vi "Helper Methods Launcher.vi"() -> ()   [LabVIEW 2020, in "2. Basic Panel Actors.lvlib"]
uses:
  2. Basic Panel Actors.lvlib
  Helper Methods/Helper Methods.lvclass
  C:/Program Files/National Instruments/LabVIEW 2020/vi.lib/MGI/Panel Manager/Panel Actor/Panel Actor/Panel Actor.lvclass
  <vilib>/MGI/Panel Manager/Panel/Window Position/Reference Position/Alignment.ctl
  <vilib>/MGI/Panel Manager/Panel/Window Position/Reference Position/Horizontal Alignment.ctl
  <vilib>/MGI/Panel Manager/Panel/Window Position/Reference Position/Vertical Alignment.ctl
  <vilib>/MGI/Panel Manager/Panel/Window Position/Reference Position/Offset/Absolute Offset/Absolute Offset.lvclass/Absolute Offset.ctl
  <vilib>/ActorFramework/Message Enqueuer/Message Enqueuer.lvclass/Message Enqueuer.ctl
  <vilib>/MGI/Panel Manager/Panel/Window Position/Reference Position/Offset/Absolute Offset/Absolute Offset.vi
  <vilib>/ActorFramework/Message Enqueuer/Enqueue.vi
  <vilib>/MGI/Panel Manager/Panel/Window Position/Reference Position/Offset/Absolute Offset/Absolute Offset.lvclass
  C:/Program Files/National Instruments/LabVIEW 2020/vi.lib/MGI/Panel Manager/Panel/Window Position/Reference Position/Offset/Offset.lvclass
  <vilib>/MGI/Panel Manager/Panel/Window Position/Reference Position/Ref VI/Ref VI.lvclass
  C:/Program Files/National Instruments/LabVIEW 2020/vi.lib/MGI/Panel Manager/Panel/Window Position/Window Position.lvclass
  <vilib>/ActorFramework/Stop Msg/Stop Msg.lvclass
  C:/Program Files/National Instruments/LabVIEW 2020/vi.lib/ActorFramework/Message/Message.lvclass
  <vilib>/MGI/Panel Manager/Panel/Window Position/Reference Position/Ref VI/Ref VI.vi
  <vilib>/MGI/Panel Manager/Panel Actor/Panel Actor/Launch Root Panel Window.vi
  <vilib>/ActorFramework/Message Priority Queue/Priority Enqueue.vi
  <vilib>/MGI/Panel Manager/Panel Actor/Panel Actor/Panel Actor.lvclass
  <vilib>/MGI/Panel Manager/Panel/Panel.lvlib
  <vilib>/MGI/Panel Manager/Panel/Window Position/Reference Position/Reference Position.lvclass
  Helper Methods Messages/Increment ID Msg/Increment ID Msg.lvclass
  C:/Program Files/National Instruments/LabVIEW 2020/vi.lib/MGI/Panel Manager/Panel/Window Position/Reference Position/Offset/Absolute Offset/Absolute Offset.lvclass
  C:/Program Files/National Instruments/LabVIEW 2020/vi.lib/MGI/Panel Manager/Panel/Window Position/Reference Position/Reference Position.lvclass
  C:/Program Files/National Instruments/LabVIEW 2020/vi.lib/MGI/Panel Manager/Panel/Window Position/Reference Position/Ref VI/Ref VI.lvclass
  C:/Program Files/National Instruments/LabVIEW 2020/vi.lib/MGI/Monitored Actor/Monitored Actor/Monitored Actor/Monitored Actor.lvclass
  C:/Program Files/National Instruments/LabVIEW 2020/vi.lib/ActorFramework/Actor/Actor.lvclass
  C:/Program Files/National Instruments/LabVIEW 2020/examples/MGI/Panel Manager/Basic Panel Actors/Helper Methods/Helper Methods/Helper Methods.lvclass
panel:
  in  "Send Increment ID":bool
  # "Run this VI to launch the Panel Actor Example.\n\nWhen the Panel Actor is running click the \"Send Increment ID\" to send the Actor a \"Increment ID\" message."
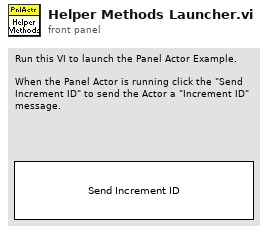
[diagram p1: front panel]
types:
  T1 = typedef "Panel.lvlib/Reference Position.lvclass/Alignment.ctl" = cluster{"Horizontal":T2, "Vertical":T3}
  T2 = typedef "Panel.lvlib/Reference Position.lvclass/Horizontal Alignment.ctl" = enum16{"Left", "Center", "Right"}
  T3 = typedef "Panel.lvlib/Reference Position.lvclass/Vertical Alignment.ctl" = enum16{"Top", "Center", "Bottom"}
  T4 = typedef "LVRectTypeDef.ctl" = cluster{"Left":i16, "Top":i16, "Right":i16, "Bottom":i16}
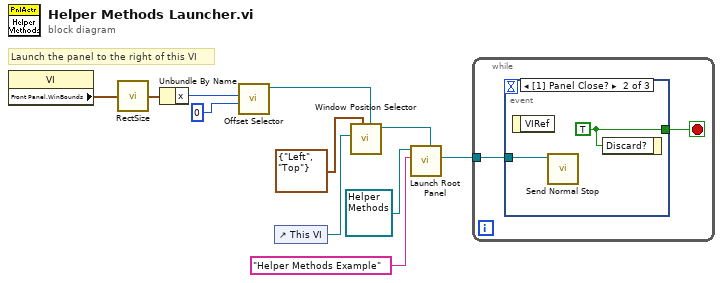
[diagram p0: block diagram]
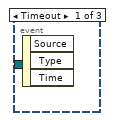
[diagram p2: hidden frame]
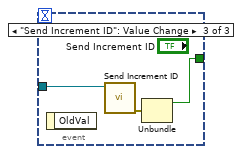
[diagram p3: hidden frame]
diagram:
  # "Launch the panel to the right of this VI"
  n1 = property class="VI"() -> ("Front Panel.WinBounds"=w5:T4)  [unwired: 2 in, 2 out]
  n2 = call <vilib>:"RectSize.vi"("rect"=w5) -> ("point"=w4:cluster{"x":i16, "y":i16})
  n3 = Unbundle By Name(w4) -> ("x"=w2:i16)
  n4 = call-poly <vilib>:"Offset Selector.vi"("Vertical"=i16 0 ("Horizontal"), "Horizontal"=w2) -> ("Absolute Offset Out"=w6:refnum<class "Absolute Offset.lvclass">)  [unwired: 8 in, 1 out]
  n5 = control-ref of="This VI"() -> (w7:refnum<vi>)
  n6 = call-poly <vilib>:"Window Position Selector.vi"("Offset"=w6, "Alignment"=T1 {"Horizontal"=enum."Left", "Vertical"=enum."Top"}, "Ref VI"=w7) -> ("Ref VI out"=w10:refnum<class "Ref VI.lvclass">)  [unwired: 7 in, 1 out]
  n7 = call-poly <vilib>:"Launch Root Panel.vi"("Window Position (Maximize First Call)"=w10, "Title"="Helper Methods Example", "Panel Actor in"=refnum<class "Helper Methods.lvclass"> refnum ("2. Basic Panel Actors.lvlib:Helper Methods.lvclass")) -> ("Actor's Enqueuer"=w3:refnum<class "Message Enqueuer.lvclass">)  [unwired: 7 in, 1 out]
  n8 = while {
    tunnel: w3 -> [w12]
    stop <- w13 stop-if-true
    n9 = event shown="[1] Panel Close?" {
      selector: _ -> [_ _ _]
      dyn-events: _ -> [_ _ _]
      timeout: _ -> [_ _ _]
      tunnel: [_ w15 w16] -> w13
      tunnel: w12 -> [_ w14 w18]
      event Timeout {
        n10 = event-data() -> ()  [unwired: 1 in, 3 out]
      }
      event Panel Close? {
        w15 = TRUE ("Discard?")
        n11 = event-data() -> ()  [unwired: 1 in, 1 out]
        n12 = call <vilib>:"Send Normal Stop.vi"("Message Enqueuer"=w14) -> ()  [unwired: 10 in, 1 out]
        n13 = event-data("Discard?"=w15) -> ()  [unwired: 1 in, 1 out]
      }
      event "Send Increment ID": Value Change {
        n14 = event-data() -> ()  [unwired: 1 in, 1 out]
        n15 = call "Send Increment ID.vi"("Message Enqueuer in"=w18) -> ("error out"=w17:errorcluster)  [unwired: 9 in, 1 out]
        n16 = Unbundle(w17) -> ("status"=w16:bool)  [unwired: 2 out]
      }
    }
  }
